vi "testSetTempObjectOrParameter.vi"() -> ()   [LabVIEW 2017]
uses:
  Common/ObjectMap/LVPortObjectMapNamepathData.ctl
  Common/ObjectMap/LVPortObjectMapDataTypeEnum.ctl
  Common/ObjectMap/LVPortObjectMapContainerTypeEnum.ctl
panel:
  in  "SomeVal":T1
  out "Object map":T2[](array[typedef])
  in  "SimpleString":string
  in  "SimpleNum":dbl
  out "pID":string
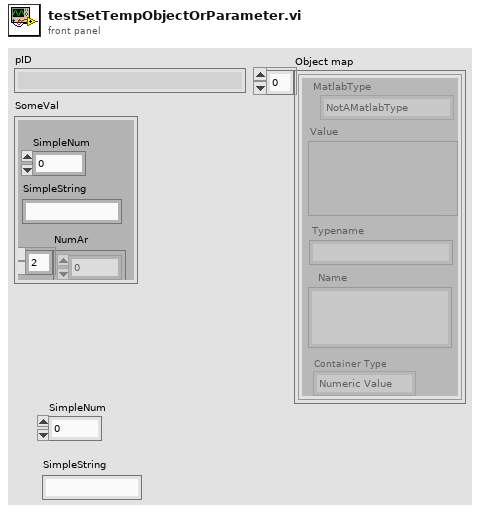
[diagram p1: front panel]
types:
  T1 = cluster{"SimpleNum":dbl, "SimpleString":string, "NumAr":dbl[]}
  T2 = typedef "LVPortObjectMapNamepathData.ctl" = cluster{"MatlabType":T3, "Value":variant, "Name":string, "Typename":string, "Container Type":T4}
  T3 = typedef "LVPortObjectMapDataTypeEnum.ctl" = enum16{"NotAMatlabType", "Real", "Complex", "String", "Boolean"}
  T4 = typedef "LVPortObjectMapContainerTypeEnum.ctl" = enum16{"Numeric Value", "Numeric Array", "Waveform"}
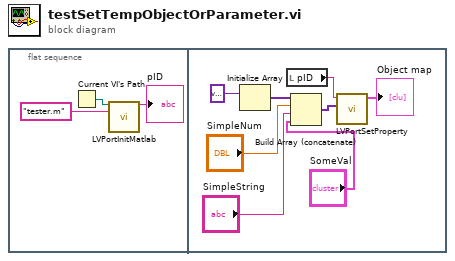
[diagram p0: block diagram]
diagram:
  n1 = flat-sequence {
    frame #0 {
      n2 = Current VI's Path() -> (path=w3:path)
      n3 = call "LVPortInitMatlab.vi"("Working directory or VI Path"=w3, "Code file name"="tester.m") -> ("ID"=→"pID":string)  [unwired: 12 in, 1 out]
    }
    frame #1 {
      n4 = Initialize Array(variant) -> (w10:variant[])  [unwired: 1 in]
      n5 = local read "pID"() -> (w7:string)
      n6 = Build Array (concatenate)(w10, "SimpleNum", "SimpleString", "SomeVal") -> (w6:variant[])
      n7 = call "LVPortSetProperty.vi"("Value"=w6, "pID"=w7) -> ("Object map"=→"Object map":T2[])  [unwired: 8 in, 1 out]
    }
  }
